vi "SLM_display_trial.vi"() -> ()   [LabVIEW 2015]
uses:
  <userlib>/TAM_Program/TAM Sub VIs.llb/BaseHologramGlobal.vi
panel:
  in  "Base hologram parameters 2":T1={"x centre A (m)"=-0.0007, "y centre A (m)"=-0.00094, "x angle A (mrad)"=0.0, "y angle A (mrad)"=10.0, "f lens A (m)"=1000000.0, "x centre B (m)"=-0.00031192399117047087, "y centre B (m)"=-0.00028507383868835634, "x angle B (mrad)"=10.0, "y angle B (mrad)"=0.0, "f lens B (m)"=1000000.0} {"f lens B (m)" format="%_3g"; "y angle B (mrad)" format="%_3g"; "x angle B (mrad)" format="%_3g"; "y centre B (m)" format="%_3p"; "x centre B (m)" format="%_3p"; "f lens A (m)" format="%_3g"; "y angle A (mrad)" format="%_3g"; "x angle A (mrad)" format="%_3g"; "y centre A (m)" format="%_3p"; "x centre A (m)" format="%_3p"}
  in  "Intensity Masking?":bool=TRUE
  in  "c":dbl
  in  "Encoding":cluster{"d":dbl, "y0":dbl, "y1":dbl}
  out "Eencoding":dbl[][](graph)
  in  "stop":bool
  in  "Load global\nbase parameters?":bool=TRUE
  in  "Base hologram parameters":T1={"x centre A (m)"=0.00023877834010536838, "y centre A (m)"=-1.0895093102686923e-05, "x angle A (mrad)"=10.0, "y angle A (mrad)"=0.0, "f lens A (m)"=1000000.0, "x centre B (m)"=-0.00031192399117047087, "y centre B (m)"=-0.00028507383868835634, "x angle B (mrad)"=10.0, "y angle B (mrad)"=0.0, "f lens B (m)"=1000000.0} {"f lens B (m)" format="%_3g"; "y angle B (mrad)" format="%_8g"; "x angle B (mrad)" format="%_8g"; "y centre B (m)" format="%_8p"; "x centre B (m)" format="%_8p"; "f lens A (m)" format="%_3g"; "y angle A (mrad)" format="%_8g"; "x angle A (mrad)" format="%_8g"; "y centre A (m)" format="%_8p"; "x centre A (m)" format="%_8p"}
  in  "beam waist w0 (m)":dbl=0.0005 format="%_3p"
  out "Hologram A":u8[][](graph)
  # "to account for \nunequal efficiencies,\nset to 1 if not intensity masking"
  # "Set global\nbase parameters?"
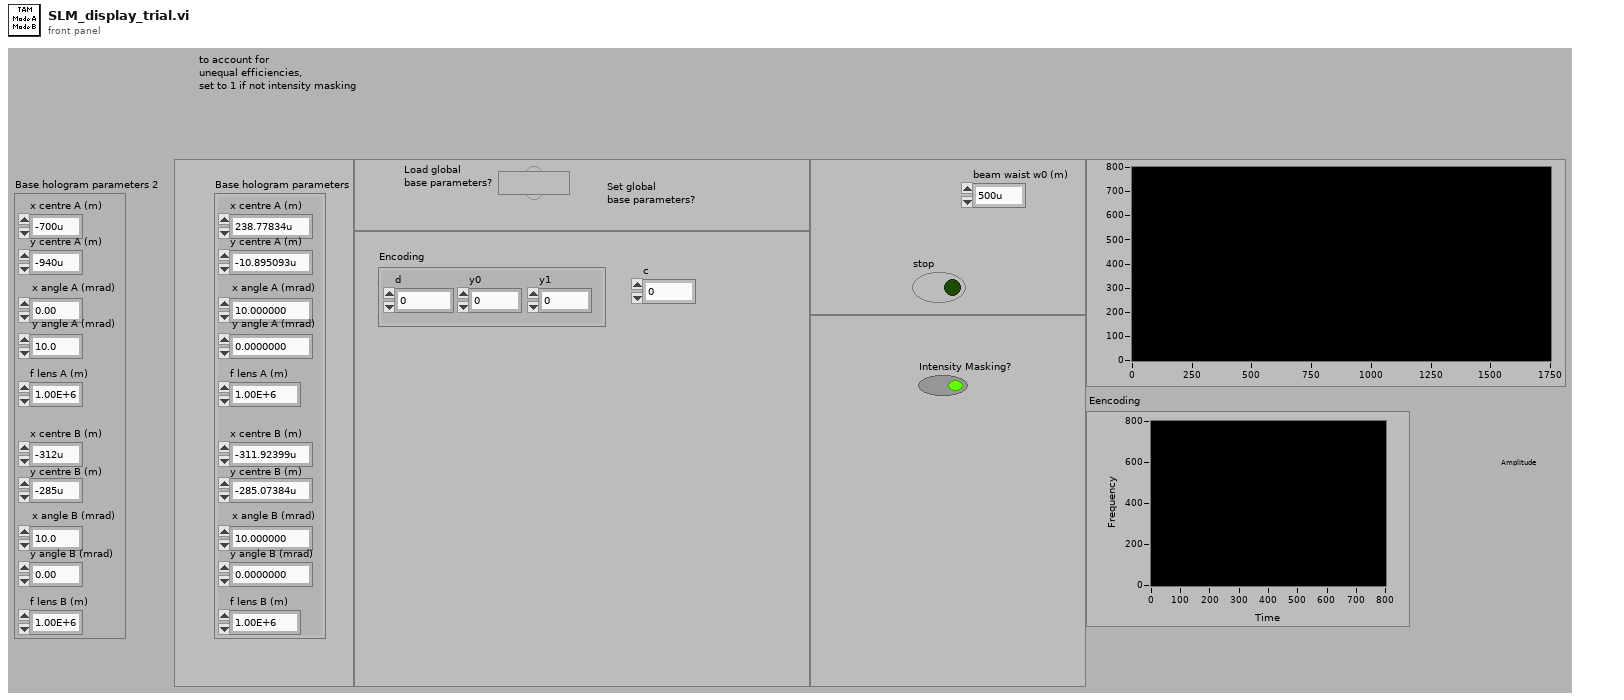
[diagram p1: front panel]
types:
  T1 = cluster{"x centre A (m)":dbl, "y centre A (m)":dbl, "x angle A (mrad)":dbl, "y angle A (mrad)":dbl, "f lens A (m)":dbl, "x centre B (m)":dbl, "y centre B (m)":dbl, "x angle B (mrad)":dbl, "y angle B (mrad)":dbl, "f lens B (m)":dbl}
  T2 = cluster{"amplitude matrix":cdb[][], "number of columns in amplitude matrix":i32, "number of rows in amplitude matrix":i32, "represented width (in m)":dbl, "represented height (in m)":dbl, "wavelength (in m)":dbl}
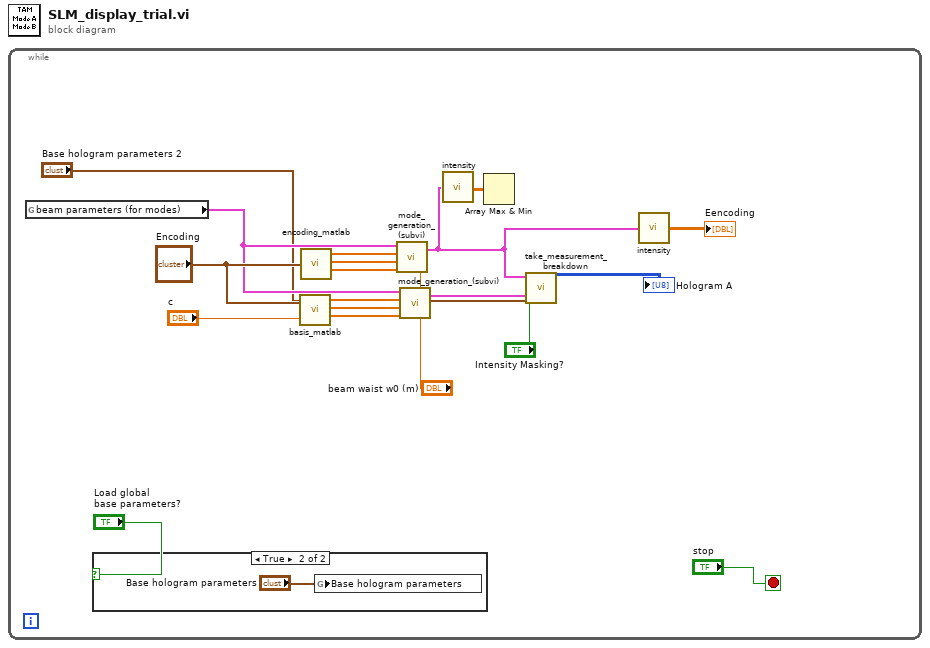
[diagram p0: block diagram]
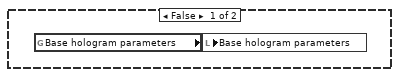
[diagram p2: hidden frame]
diagram:
  n1 = while {
    stop <- "stop" stop-if-true
    n2 = global read "BaseHologramGlobal.vi" "beam parameters (for modes)"() -> (w4:T2)
    n3 = case shown="True" "Load global\nbase parameters?" {
      frame False {
        n4 = global read "BaseHologramGlobal.vi" "Base hologram parameters"() -> (w20:T1)
        n5 = local write "Base hologram parameters"(w20) -> ()
      }
      frame True {
        n6 = global write "BaseHologramGlobal.vi" "Base hologram parameters"("Base hologram parameters") -> ()
      }
    }
    n7 = call "basis_matlab.vi"("Encoding"="Encoding", "c"="c") -> ("modes"=w12:dbl[], "coeffs"=w11:dbl[], "phases"=w10:dbl[])
    n8 = call "encoding_matlab.vi"("Encoding"="Encoding") -> ("modes"=w9:dbl[], "coeffs"=w8:dbl[], "phase"=w7:dbl[])
    n9 = call "mode_generation_(subvi).vi"("beam waist w0 (m) in"="beam waist w0 (m)", "phase"=w7, "coeffs"=w8, "modes"=w9, "beam parameters in"=w4) -> ("mode encoding"=w14:T2)
    n10 = call "mode_generation_(subvi).vi"("beam waist w0 (m) in"="beam waist w0 (m)", "phase"=w10, "coeffs"=w11, "modes"=w12, "beam parameters in"=w4) -> ("mode encoding"=w3:T2)
    n11 = call <userlib>:"intensity.vi"("beam cluster"=w14) -> ("intensity matrix"=w16:dbl[][])
    n12 = Array Max & Min(array=w16) -> ()  [unwired: 4 out]
    n13 = call "take_measurement_breakdown.vi"("Base hologram parameters"="Base hologram parameters 2", "Intensity Masking?"="Intensity Masking?", "Mode B"=w3, "Mode A"=w14) -> ("Hologram"=→"Hologram A":u8[][])  [unwired: 7 in]
    n14 = call <userlib>:"intensity.vi"("beam cluster"=w14) -> ("intensity matrix"=→"Eencoding":dbl[][])
  }
